vi "ADS1015_Current_Monitoring.vi"() -> ()   [LabVIEW 2018]
uses:
  <vilib>/MakerHub/LINX/Private/Device/Type Defs/TCP Config.ctl
  User Defined/I2C_Platform_Selector.ctl
  <vilib>/MakerHub/LINX/Public/Utilities/Open TCP.vi
  <vilib>/MakerHub/LINX/LMH-LINX.lvlib
  <vilib>/MakerHub/LINX/Private/Device/Device.lvlib
panel:
  out "Offset":dbl
  in  "Calib":bool
  out "New value":dbl format="%#_3g"
  in  "SCAN IP":bool
  in  "Range":T1(ring)
  out "Current":dbl caption="mA" format="%#_3g"
  in  "PAUSE":bool
  in  "Start":bool
  out "output waveform":waveform(dbl)
  out "Waveform Chart":waveform(dbl)(graph)
  in  "App_Stop":bool
  in  "TCP Configuration":T2={"IP Address"="192.168.1.5", "Port"=44300}
  in  "Acquire":bool
  # "Wireless DC POWER Analyzer"
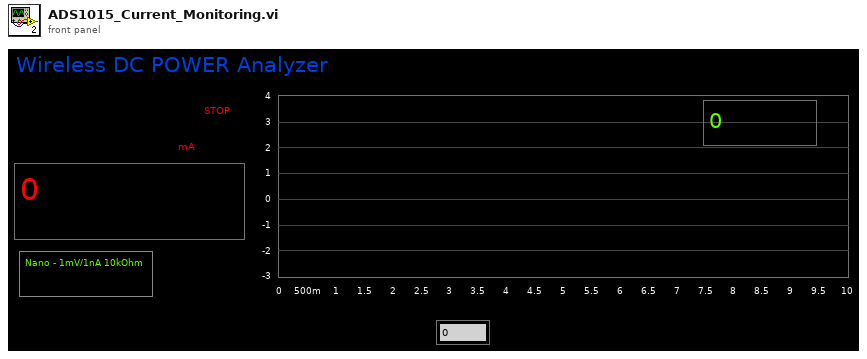
[diagram p1: front panel]
types:
  T1 = enum16{"Nano - 1mV/1nA 10kOhm", "Micro - 1mV/1uA 10Ohm", "Mili  -  1mV/1mA 0.01Ohm"}
  T2 = typedef "LMH-LINX.lvlib/Device.lvlib/TCP Config.ctl" = cluster{"IP Address":string, "Port":u16}
  T3 = typedef "I2C_Platform_Selector.ctl" = enum16{"ESP8266-I2C", "Raspberry Pi-I2C"}
  T4 = cluster{"ADS1015-Channel Selector":enum8{"DIFF-AI0-AI1", "DIFF-AI0-AI3", "DIFF-AI1-AI3", "DIFF-AI2-AI3", "Single Ended - AI0", "Single Ended - AI1", "Single Ended - AI2", "Single Ended - AI3"}, "ADS1015 -Gain & Scale":enum8{"FS=+/-6.144 V", "FS=+/-4.096 V", "FS=+/-2.048 V", "FS=+/-1.024 V", "FS=+/-0.512 V", "FS=+/-0.256-A V", "FS=+/-0.256-B V", "FS=+/-0.256-C V"}, "ADS1015- Acquire Mode":enum16{"Continuous Conversion Mode", "Single Shot Mode"}, "ADS1015 Sample Rate":enum8{"128 SPS", "250 SPS", "490 SPS", "920 SPS", "1600 SPS", "2400 SPS", "3300 SPS", "3300 SPS A"}}
  T5 = typedef "LMH-LINX.lvlib/LINX Ref.ctl" = cluster{"IO":T6, "Interface":T7, "LINX Device Config":T8}
  T6 = typedef "LMH-LINX.lvlib/Platform.ctl" = enum16{"Remote", "Local"}
  T7 = typedef "LMH-LINX.lvlib/Interface.ctl" = enum16{"Serial", "TCP"}
  T8 = typedef "LMH-LINX.lvlib/Device.lvlib/LINX Device Config.ctl" = cluster{"Interface":T7, "COM Port":refnum<visa-resource-name>, "TCP Configuration":T2, "Device Family":u8, "Device ID":u8, "Device Name":string, "TCP Ref":refnum<k5>, "Channels":T9}
  T9 = typedef "LMH-LINX.lvlib/Channels.ctl" = cluster{"DI":u8[], "DO":u8[], "AI":u8[], "AO":u8[], "PWM":u8[], "QE":u8[], "UART":u8[], "I2C 2":u8[], "SPI":u8[], "CAN":u8[], "Servo":u8[], "AI Ref (V)":dbl, "AI Resolution (Bits)":u8, "AO Ref (V)":dbl, "AO Resolution (Bits)":u8}
  T10 = enum8{"FS=+/-6.144 V", "FS=+/-4.096 V", "FS=+/-2.048 V", "FS=+/-1.024 V", "FS=+/-0.512 V", "FS=+/-0.256-A V", "FS=+/-0.256-B V", "FS=+/-0.256-C V"}
  T11 = enum8{"DIFF-AI0-AI1", "DIFF-AI0-AI3", "DIFF-AI1-AI3", "DIFF-AI2-AI3", "Single Ended - AI0", "Single Ended - AI1", "Single Ended - AI2", "Single Ended - AI3"}
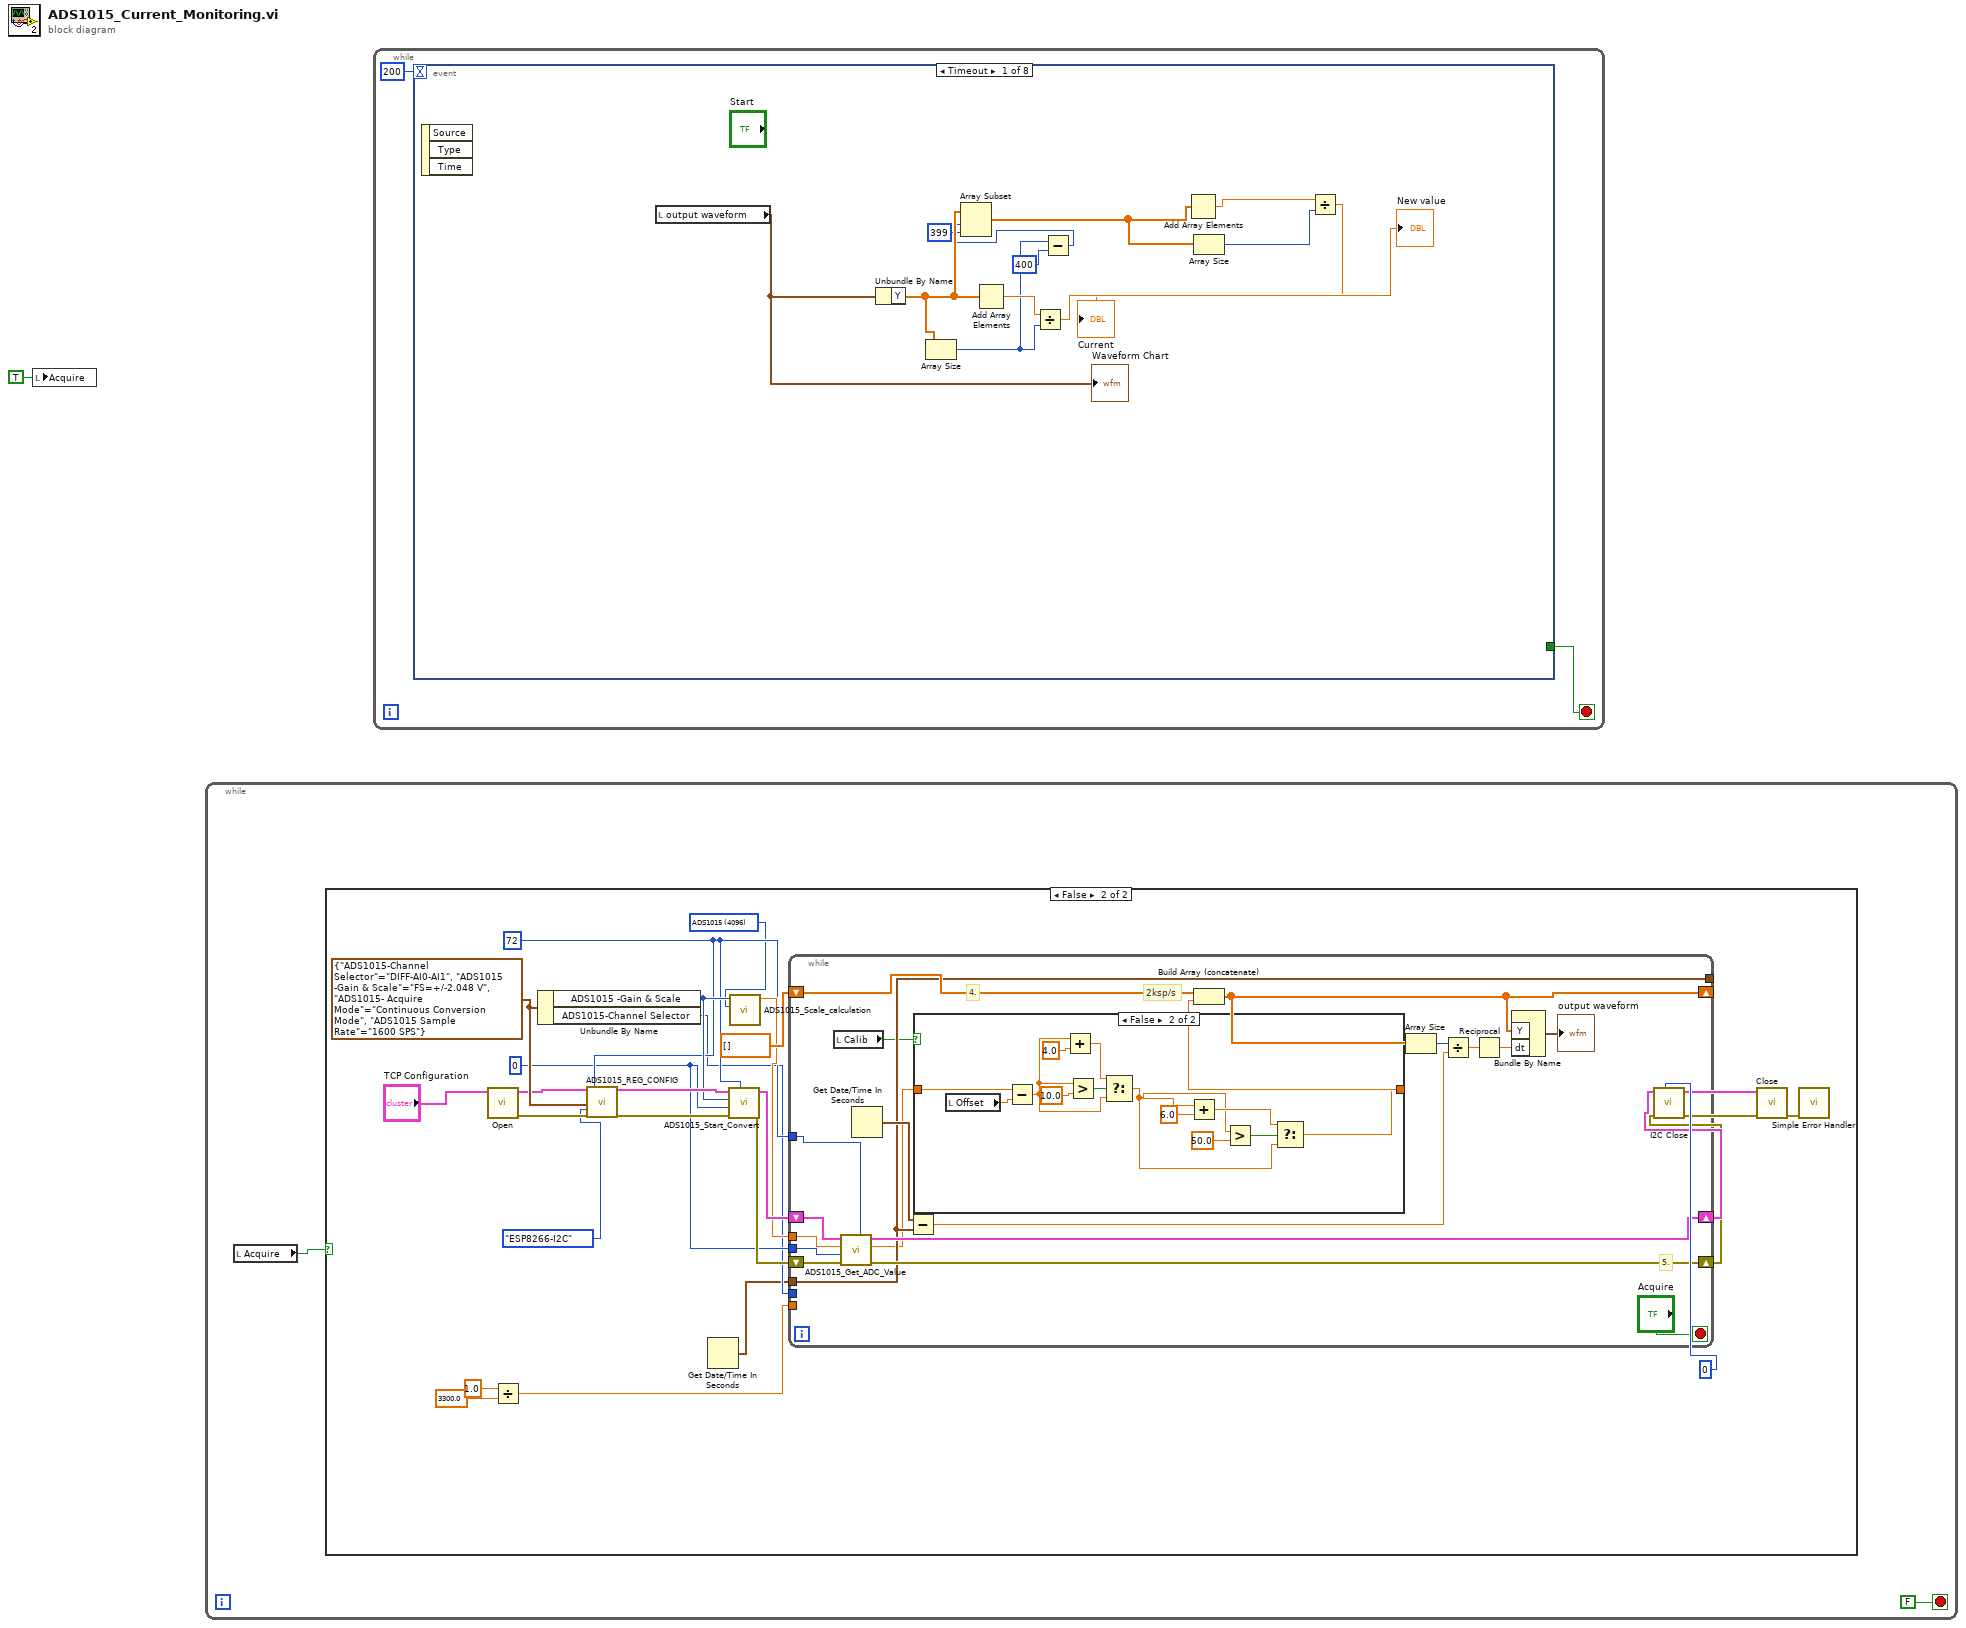
[diagram p0: block diagram]
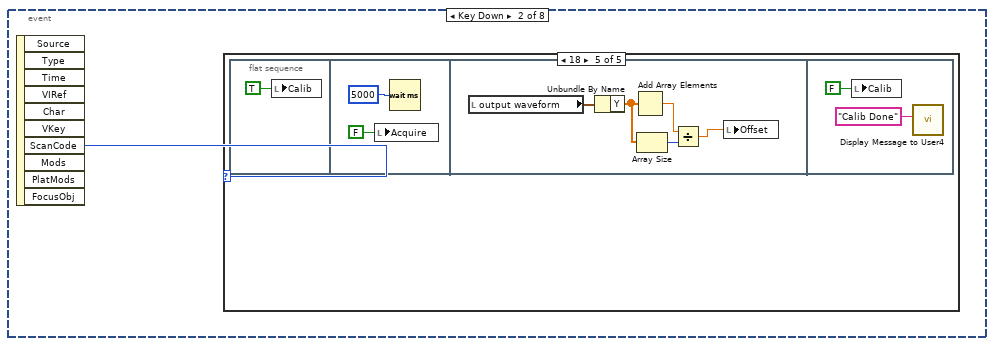
[diagram p4: hidden frame]
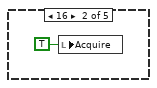
[diagram p6: hidden frame]
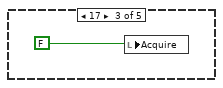
[diagram p7: hidden frame]
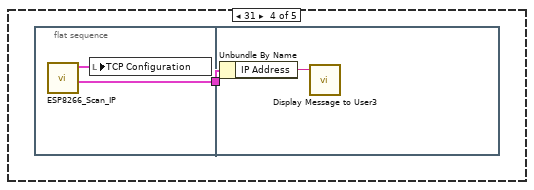
[diagram p8: hidden frame]
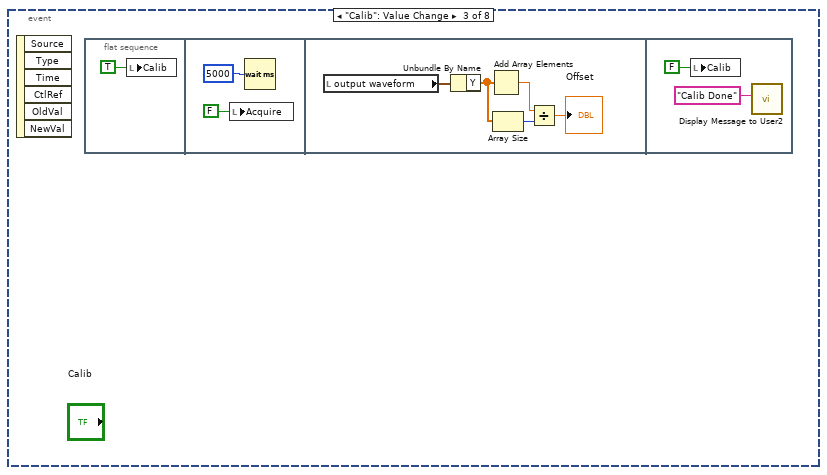
[diagram p9: hidden frame]
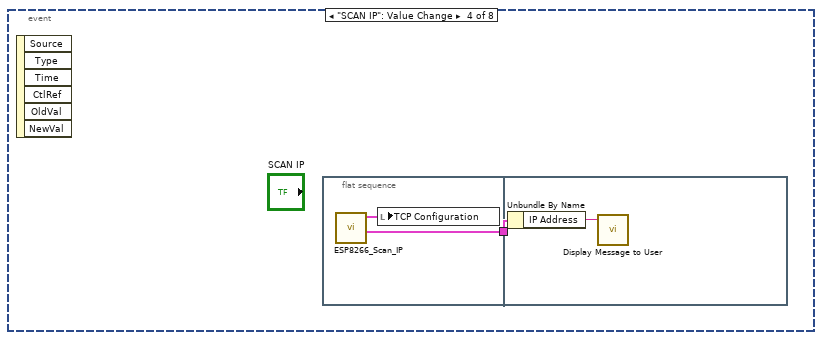
[diagram p10: hidden frame]
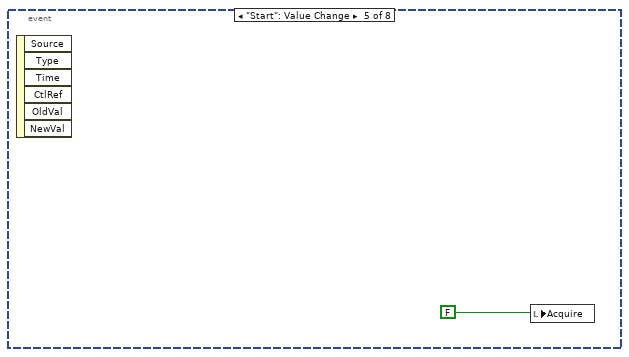
[diagram p11: hidden frame]
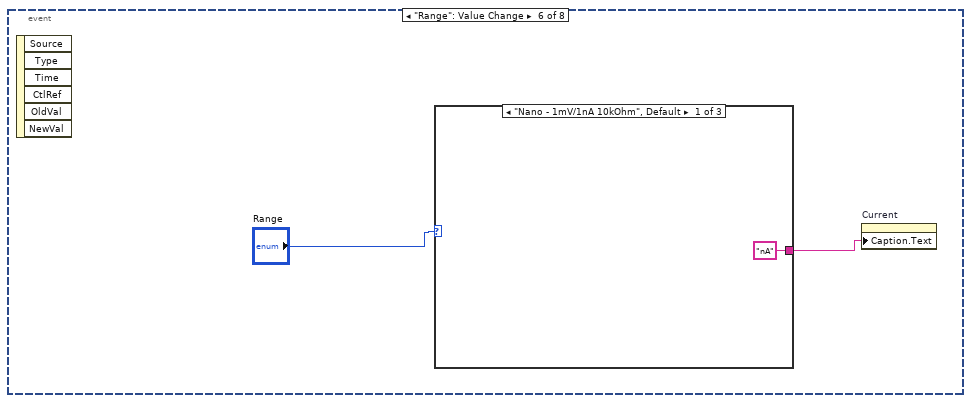
[diagram p12: hidden frame]
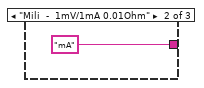
[diagram p13: hidden frame]
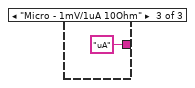
[diagram p14: hidden frame]
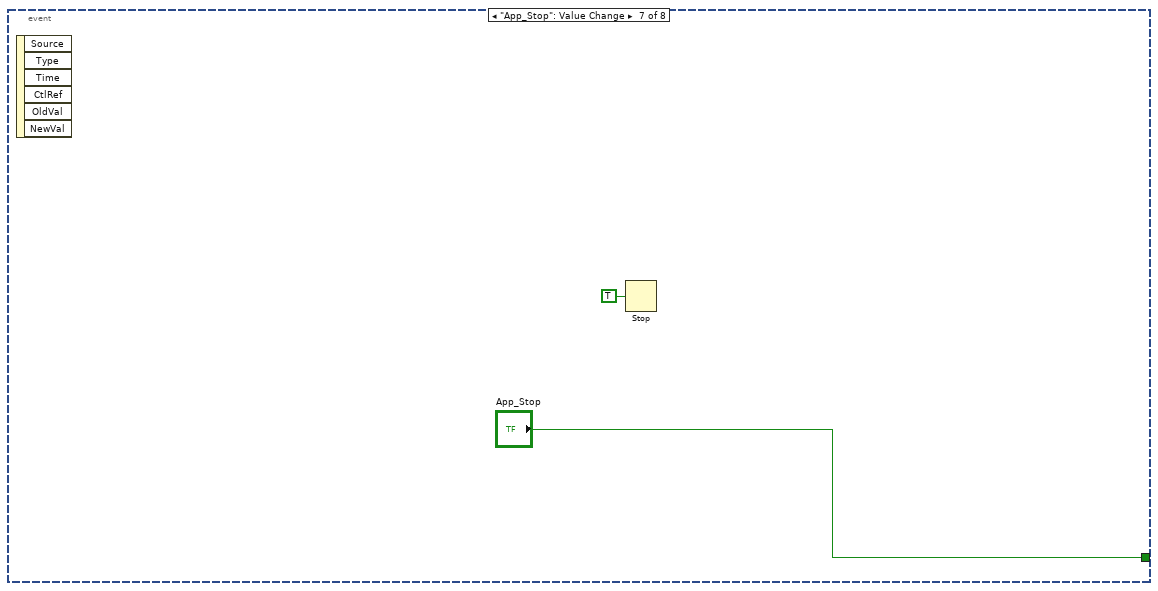
[diagram p15: hidden frame]
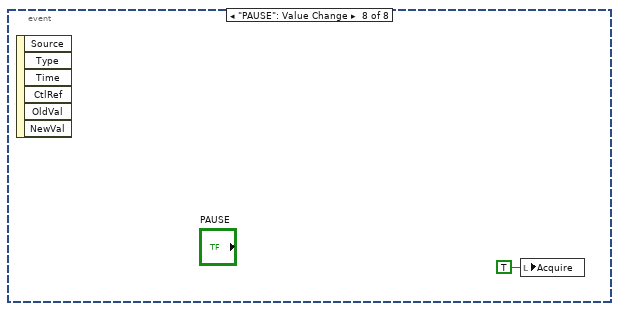
[diagram p16: hidden frame]
diagram:
  n1 = local write "Acquire"(TRUE ("Acquire")) -> ()
  n2 = while {
    stop <- FALSE stop-if-true
    n3 = local read "Acquire"() -> (w3:bool)
    n4 = case shown="False" w3 {
      frame True {
      }
      frame False {
        w9 = 4096 items=["ADS1015"=4096, "AD1115"=65536] ("IC Selector")
        w11 = u8 0 ("I2C Channel (RPI)")
        w13 = u8 72 ("I2C Slave Address (0)")
        w22 = T4 {"ADS1015-Channel Selector"=enum."DIFF-AI0-AI1", "ADS1015 -Gain & Scale"=enum."FS=+/-2.048 V", "ADS1015- Acquire Mode"=enum."Continuous Conversion Mode", "ADS1015 Sample Rate"=enum."1600 SPS"} ("ADS1015 Reg Config")
        n5 = call-poly <vilib>:"Open.vi"("TCP Configuration"="TCP Configuration") -> ("Error Out"=w14:errorcluster, "LINX Resource"=w15:T5)  [unwired: 8 in, 1 out]
        n6 = Divide(x=1.0, y=3300.0) -> (x/y=w5:dbl)
        n7 = Unbundle By Name(w22) -> ("ADS1015 -Gain & Scale"=w21:T10, "ADS1015-Channel Selector"=w8:T11)
        n8 = call "ADS1015_REG_CONFIG.vi"("LINX Resource in"=w15, "ADS1015 Reg Config"=w22, "I2C_Channel_platform"=I2C_Platform_Selector."ESP8266-I2C", "Error In"=w14, "I2C Slave Address (0)"=w13) -> ("LINX Resource out"=w25:T5, "Error Out"=w28:errorcluster)  [unwired: 13 in]
        n9 = Get Date/Time In Seconds() -> (seconds since 1Jan1904=w4:timestamp)
        n10 = call "ADS1015_Start_Convert.vi"("I2C Slave Address (0)"=w13, "error in (no error)"=w28, "I2C_Channel_platform"=w11, "Scale mV"=w21, "LINX Resource in"=w25) -> ("error out"=w27:errorcluster, "LINX Resource out"=w24:T5)  [unwired: 4 in, 1 out]
        n11 = call "ADS1015_Scale_calculation.vi"("IC Selector"=w9, "ADS1015 -Gain & Scale"=w21) -> ("Scale Value (mV)"=w23:dbl)  [unwired: 9 in]
        n12 = while {
          shift-right: [w45] -> w19
          shift-left: w24 -> [w46]
          shift-right: [w49] -> w17
          shift-left: w27 -> [w48]
          shift-right: [w38] -> _
          shift-left: dbl[] [] -> [w47]
          tunnel: w13 -> [w44]
          tunnel: w23 -> [w41]
          tunnel: w11 -> [w42]
          tunnel: w8 -> [_]
          tunnel: w5 -> [_]
          tunnel: w4 -> [w39]
          tunnel: [w39] -> _
          stop <- "Acquire" stop-if-true
          # "2ksp/s"
          # "5."
          # "4."
          n13 = local read "Calib"() -> (w30:bool)
          n14 = call "ADS1015_Get_ADC_Value.vi"("I2C Slave Address (0)"=w44, "error in (no error)"=w48, "I2C_Channel_platform"=w42, "Scale Value (mV)"=w41, "LINX Resource in"=w46) -> ("error out"=w49:errorcluster, "mV out"=w32:dbl, "LINX Resource"=w45:T5)  [unwired: 3 in, 1 out]
          n15 = Get Date/Time In Seconds() -> (seconds since 1Jan1904=w40:timestamp)
          n16 = Subtract(x=w40, y=w39) -> (x-y=w36:dbl)
          n17 = case shown="False" w30 {
            tunnel: w32 -> [w50 w63]
            tunnel: [w50 w51] -> w31
            frame True {
            }
            frame False {
              n18 = local read "Offset"() -> (w62:dbl)
              n19 = Subtract(x=w63, y=w62) -> (x-y=w57:dbl)
              n20 = Add(x=w57, y=4.0) -> (x+y=w58:dbl)
              n21 = Greater?(x=w57, y=10.0) -> (0:w60:bool)
              n22 = Select(t=w58, s=w60, f=w57) -> (s? t:f=w52:dbl)
              n23 = Add(x=w52, y=6.0) -> (x+y=w53:dbl)
              n24 = Greater?(x=w52, y=50.0) -> (0:w54:bool)
              n25 = Select(t=w53, s=w54, f=w52) -> (s? t:f=w51:dbl)
            }
          }
          n26 = Build Array (concatenate)(w47, w31) -> (w38:dbl[])
          n27 = Array Size(array=w38) -> (size(s)=w37:i32)
          n28 = Divide(x=w37, y=w36) -> (x/y=w35:dbl)
          n29 = Reciprocal(x=w35) -> (1/x=w34:dbl)
          n30 = Bundle By Name("Y"=w38, "dt"=w34) -> (→"output waveform":waveform(dbl))  [unwired: 1 in]
        }
        n31 = call <vilib>:"I2C Close.vi"("I2C Channel (0)"=u8 0, "Error In"=w17, "LINX Resource"=w19) -> ("Error Out"=w16:errorcluster, "LINX Resource"=w18:T5)  [unwired: 7 in]
        n32 = call <vilib>:"Close.vi"("Error In"=w16, "LINX Resource"=w18) -> ("Error Out"=w29:errorcluster)  [unwired: 9 in]
        n33 = call <vilib>:"Simple Error Handler.vi"("error in (no error)"=w29) -> ()  [unwired: 4 in, 5 out]
      }
    }
  }
  n34 = while {
    stop <- w65 stop-if-true
    n35 = event shown="[0] Timeout" {
      selector: _ -> [_ _ _ _ _ _ _ _]
      dyn-events: _ -> [_ _ _ _ _ _ _ _]
      timeout: 200 -> [_ _ _ _ _ _ _ _]
      tunnel: [_ _ _ _ _ _ "App_Stop" _] -> w65
      event Timeout {
        n36 = event-data() -> ()  [unwired: 1 in, 3 out]
        n37 = local read "output waveform"() -> (w77:waveform(dbl))
        "Waveform Chart" <- w77
        n38 = Unbundle By Name(w77) -> ("Y"=w75:dbl[])
        n39 = Array Size(array=w75) -> (size(s)=w74:i32)
        n40 = Add Array Elements(numeric array=w75) -> (sum=w76:dbl)
        n41 = Divide(x=w76, y=w74) -> (x/y=→"New value":dbl)
        n42 = Subtract(x=w74, y=400) -> (x-y=w72:i32)
        n43 = Array Subset(array=w75, index=w72, length=399) -> (w70:dbl[])
        n44 = Add Array Elements(numeric array=w70) -> (sum=w69:dbl)
        n45 = Array Size(array=w70) -> (size(s)=w68:i32)
        n46 = Divide(x=w69, y=w68) -> (x/y=→"Current":dbl)
      }
      event Key Down {
        n47 = event-data() -> ("ScanCode"=w78:i16)  [unwired: 1 in, 9 out]
        n48 = case shown="18" w78 {
          frame 0, Default {
          }
          frame 16 {
            n49 = local write "Acquire"(TRUE ("Acquire")) -> ()
          }
          frame 17 {
            n50 = local write "Acquire"(FALSE) -> ()
          }
          frame 31 {
            n51 = flat-sequence {
              tunnel: [w82] -> w81
              tunnel: w81 -> [w84]
              frame #0 {
                n52 = call "ESP8266_Scan_IP.vi"() -> ("TCP Configuration"=w82:T2)  [unwired: 11 in]
                n53 = local write "TCP Configuration"(w82) -> ()
              }
              frame #1 {
                n54 = Unbundle By Name(w84) -> ("IP Address"=w83:string)
                n55 = call "Display Message to User3"("Message"=w83) -> ()  [unwired: 9 in, 2 out]
              }
            }
          }
          frame 18 {
            n56 = flat-sequence {
              frame #0 {
                n57 = local write "Calib"(TRUE ("Calib")) -> ()
              }
              frame #1 {
                n58 = local write "Acquire"(FALSE) -> ()
                n59 = Wait (ms)(milliseconds to wait=u32 5000) -> ()  [unwired: 1 out]
              }
              frame #2 {
                n60 = local read "output waveform"() -> (w89:waveform(dbl))
                n61 = Unbundle By Name(w89) -> ("Y"=w91:dbl[])
                n62 = Add Array Elements(numeric array=w91) -> (sum=w92:dbl)
                n63 = Array Size(array=w91) -> (size(s)=w90:i32)
                n64 = Divide(x=w92, y=w90) -> (x/y=w88:dbl)
                n65 = local write "Offset"(w88) -> ()
              }
              frame #3 {
                n66 = local write "Calib"(FALSE ("Calib")) -> ()
                n67 = call "Display Message to User4"("Message"="Calib Done") -> ()  [unwired: 9 in, 2 out]
              }
            }
          }
        }
      }
      event "Calib": Value Change {
        n68 = event-data() -> ()  [unwired: 1 in, 6 out]
        n69 = flat-sequence {
          frame #0 {
            n70 = local write "Calib"(TRUE ("Calib")) -> ()
          }
          frame #1 {
            n71 = local write "Acquire"(FALSE) -> ()
            n72 = Wait (ms)(milliseconds to wait=u32 5000) -> ()  [unwired: 1 out]
          }
          frame #2 {
            n73 = local read "output waveform"() -> (w99:waveform(dbl))
            n74 = Unbundle By Name(w99) -> ("Y"=w101:dbl[])
            n75 = Add Array Elements(numeric array=w101) -> (sum=w102:dbl)
            n76 = Array Size(array=w101) -> (size(s)=w100:i32)
            n77 = Divide(x=w102, y=w100) -> (x/y=→"Offset":dbl)
          }
          frame #3 {
            n78 = local write "Calib"(FALSE ("Calib")) -> ()
            n79 = call "Display Message to User2"("Message"="Calib Done") -> ()  [unwired: 9 in, 2 out]
          }
        }
      }
      event "SCAN IP": Value Change {
        n80 = event-data() -> ()  [unwired: 1 in, 6 out]
        n81 = flat-sequence {
          tunnel: [w106] -> w105
          tunnel: w105 -> [w108]
          frame #0 {
            n82 = call "ESP8266_Scan_IP.vi"() -> ("TCP Configuration"=w106:T2)  [unwired: 11 in]
            n83 = local write "TCP Configuration"(w106) -> ()
          }
          frame #1 {
            n84 = Unbundle By Name(w108) -> ("IP Address"=w107:string)
            n85 = call "Display Message to User"("Message"=w107) -> ()  [unwired: 9 in, 2 out]
          }
        }
      }
      event "Start": Value Change {
        n86 = event-data() -> ()  [unwired: 1 in, 6 out]
        n87 = local write "Acquire"(FALSE) -> ()
      }
      event "Range": Value Change {
        n88 = event-data() -> ()  [unwired: 1 in, 6 out]
        n89 = case shown="\"Nano - 1mV/1nA 10kOhm\", Default" "Range" {
          tunnel: ["nA" "mA" "uA"] -> w110
          frame "Nano - 1mV/1nA 10kOhm", Default {
          }
          frame "Mili  -  1mV/1mA 0.01Ohm" {
          }
          frame "Micro - 1mV/1uA 10Ohm" {
          }
        }
        n90 = property on="Current" class="DigNum (strict)"("Caption.Text"=w110) -> ()  [unwired: 2 in, 2 out]
      }
      event "App_Stop": Value Change {
        n91 = event-data() -> ()  [unwired: 1 in, 6 out]
        n92 = Stop(stop? (T)=TRUE) -> ()
      }
      event "PAUSE": Value Change {
        n93 = event-data() -> ()  [unwired: 1 in, 6 out]
        n94 = local write "Acquire"(TRUE ("Acquire")) -> ()
      }
    }
  }
